vi "Curcular Buffer Data History.vi"(6 "Oldest time to Plot":dbl, 7 "write (F)":bool, 8 "Error In":errorcluster, 9 "Data Value":dbl, 10 "Time Stamp":dbl format="%^<%H:%M:%S%4u\n%x>T", 11 "Device Name":string) -> (0 "Error Out":errorcluster, 1 "Latest Timestamp":dbl, 2 "Latest Value":dbl, 3 "Truncated Data History":T1)   [LabVIEW 2014]
uses:
  typedefs/DVR Map Action.ctl
  typedefs/Data History.ctl
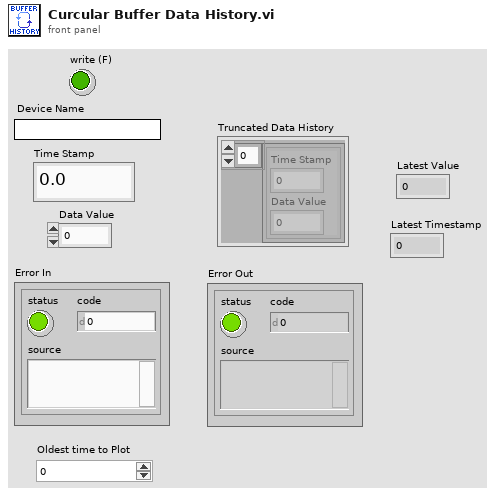
[diagram p1: front panel]
types:
  T1 = cluster{cluster{"Time Stamp":dbl, "Data Value":dbl}[]}
  T2 = typedef "DVR Map Action.ctl" = enum16{"Read Names", "Write", "Read"}
  T3 = typedef "Data History.ctl" = cluster{"Timestamps":dbl[], "Values":dbl[]}
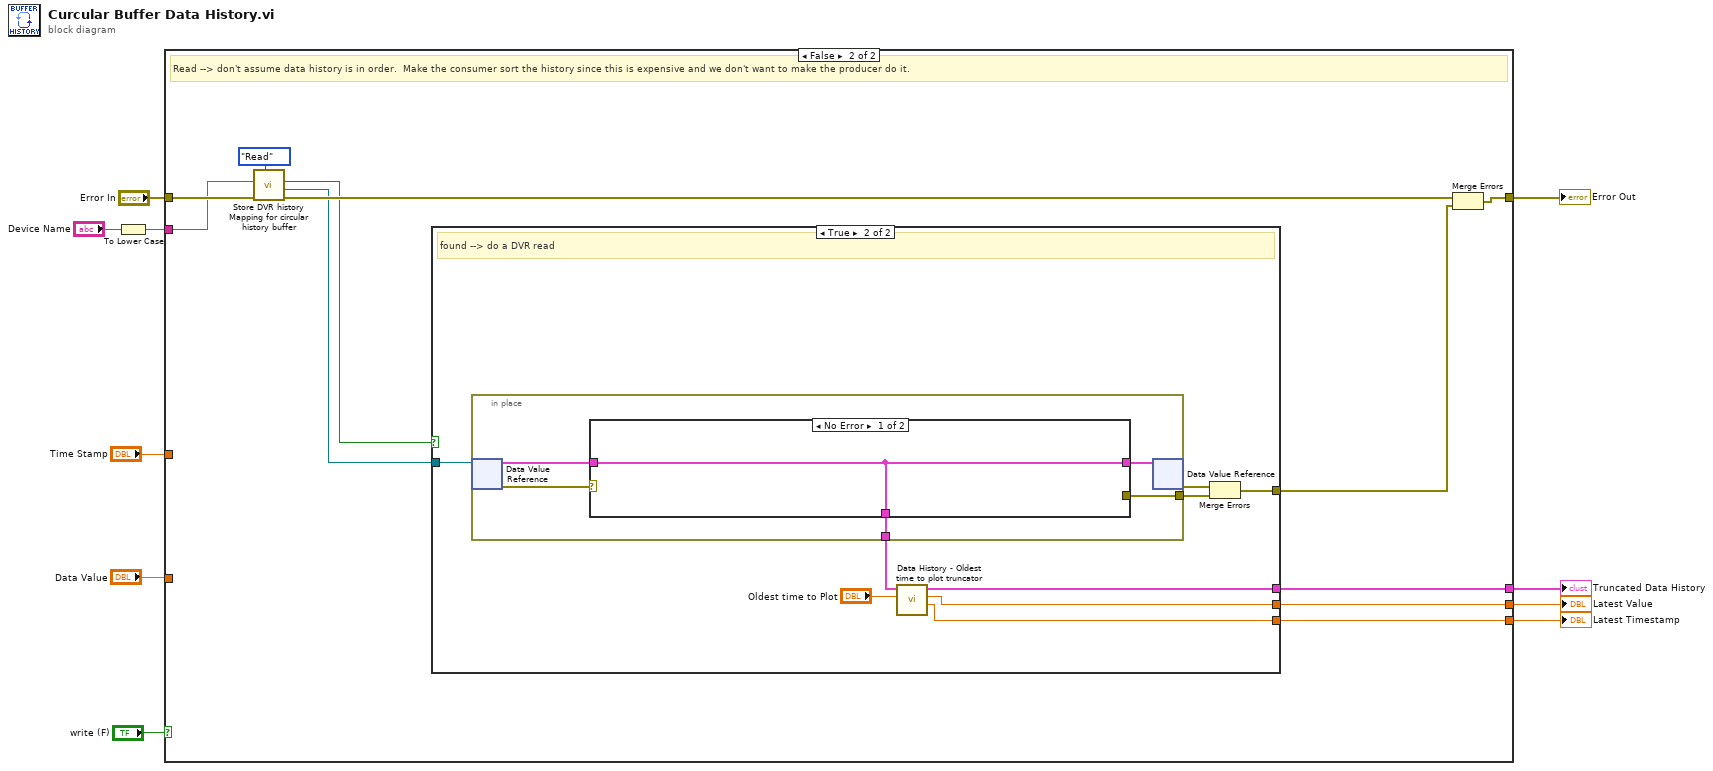
[diagram p0: block diagram]
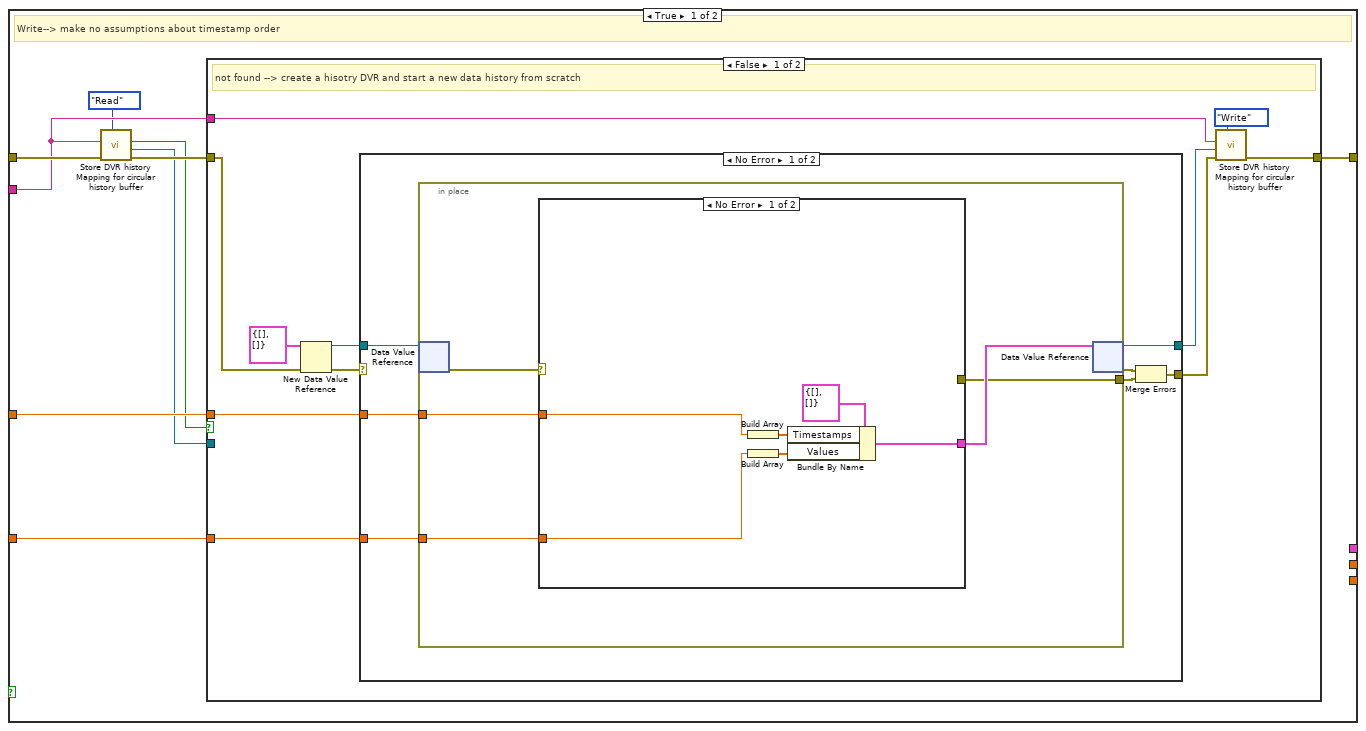
[diagram p2: hidden frame]
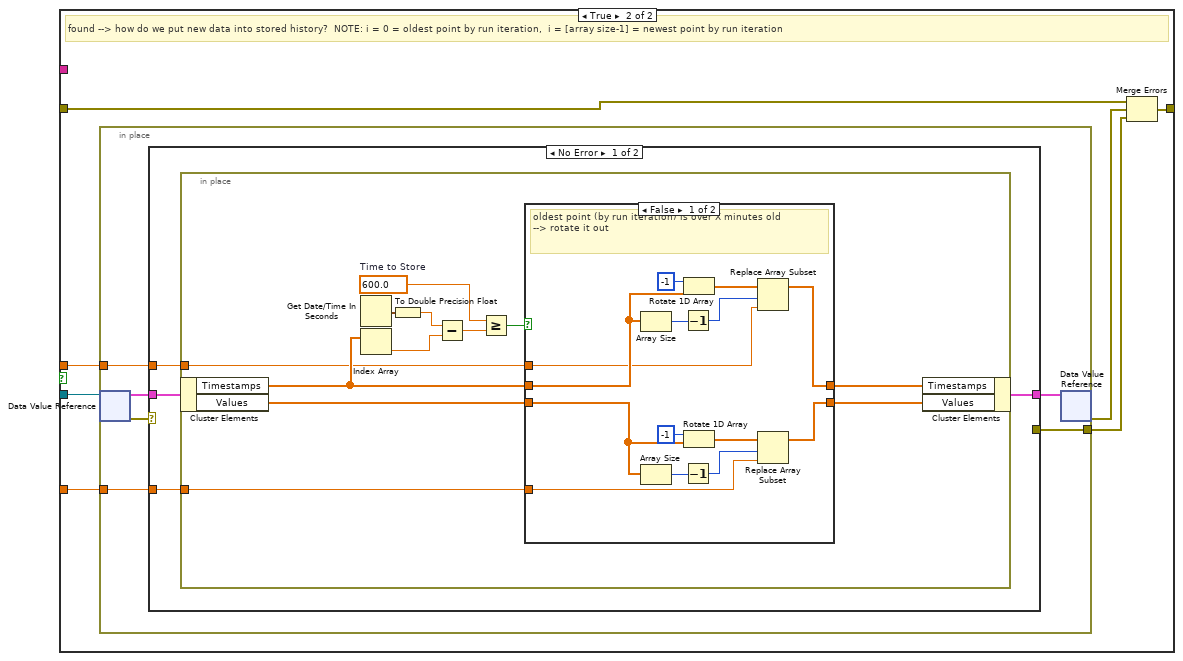
[diagram p5: hidden frame]
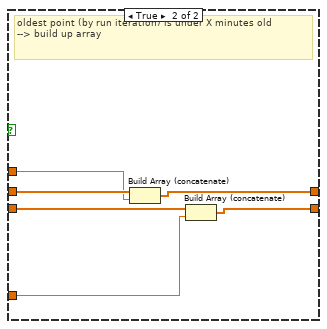
[diagram p6: hidden frame]
diagram:
  n1 = To Lower Case(string="Device Name") -> (all lower case string=w2:string)
  n2 = case shown="False" "write (F)" {
    tunnel: w2 -> [w12 w102]
    tunnel: "Time Stamp" -> [w19 _]
    tunnel: "Data Value" -> [w18 _]
    tunnel: [w17 w110] -> w6
    tunnel: "Error In" -> [w16 w106]
    tunnel: [_ w109] -> w3
    tunnel: [_ w108] -> w5
    tunnel: [_ w107] -> w4
    frame True {
      # "Write--> make no assumptions about timestamp order"
      n3 = call "Store DVR history Mapping for circular history buffer.vi"("Action"=DVR_Map_Action."Read", "error in"=w16, "Device Name"=w12) -> ("error out"=w15:errorcluster, "History DVR"=w13:refnum<data-value>, "Found?"=w14:bool)  [unwired: 5 in, 1 out]
      n4 = case shown="False" w14 {
        tunnel: w13 -> [_ w55]
        tunnel: w19 -> [w30 w57]
        tunnel: w18 -> [w29 w56]
        tunnel: w12 -> [w21 _]
        tunnel: w15 -> [w26 w51]
        tunnel: [w23 w54] -> w17
        frame False {
          # "not found --> create a hisotry DVR and start a new data history from scratch"
          n5 = New Data Value Reference(data value=T3 {"Timestamps"=[], "Values"=[]} ("Current Value Data"), error in=w26) -> (data value reference=w27:refnum<data-value>, error out=w25:errorcluster)
          n6 = case shown="No Error" w25 {
            selector: w25 -> [_ w50]
            tunnel: w30 -> [w37 _]
            tunnel: w29 -> [w36 _]
            tunnel: w27 -> [w35 _]
            tunnel: [w32 w50] -> w24
            tunnel: [w31 _] -> w22
            frame No Error {
              n7 = in-place {
                in-place-border: w37 -> [w42]
                in-place-border: w36 -> [w41]
                in-place-border: [w38] -> w33
                n8 = in-place-dvr #1(w35) -> (w40:errorcluster)  [unwired: 1 out]
                n9 = case shown="No Error" w40 {
                  selector: w40 -> [_ w49]
                  tunnel: w42 -> [w47 _]
                  tunnel: w41 -> [w46 _]
                  tunnel: [w43 _] -> w39
                  tunnel: [_ w49] -> w38
                  frame No Error {
                    n10 = Build Array(w47) -> (w45:dbl[])
                    n11 = Build Array(w46) -> (w44:dbl[])
                    n12 = Bundle By Name(cluster=T3 {"Timestamps"=[], "Values"=[]} ("Current Value Data"), "Timestamps"=w45, "Values"=w44) -> (w43:T3)
                  }
                  frame Error {
                  }
                }
                n13 = in-place-dvr #1(w39) -> (w31:refnum<data-value>, w34:errorcluster)
              }
              n14 = Merge Errors(w34, w33) -> (w32:errorcluster)
            }
            frame Error {
            }
          }
          n15 = call "Store DVR history Mapping for circular history buffer.vi"("Action"=DVR_Map_Action."Write", "error in"=w24, "History DVR"=w22, "Device Name"=w21) -> ("error out"=w23:errorcluster)  [unwired: 4 in, 3 out]
        }
        frame True {
          # "found --> how do we put new data into stored history?  NOTE: i = 0 = oldest point by run iteration,  i = [array size-1] = newest point by run iteration"
          n16 = in-place {
            in-place-border: w57 -> [w62]
            in-place-border: w56 -> [w63]
            in-place-border: [w58] -> w53
            n17 = in-place-dvr #2(w55) -> (w60:T3, w61:errorcluster)
            n18 = case shown="No Error" w61 {
              selector: w61 -> [_ w100]
              tunnel: w63 -> [w67 _]
              tunnel: w62 -> [w66 _]
              tunnel: w60 -> [w65 _]
              tunnel: [w64 _] -> w59
              tunnel: [_ w100] -> w58
              frame No Error {
                n19 = in-place {
                  in-place-border: w67 -> [w79]
                  in-place-border: w66 -> [w73]
                  w71 = 600.0  # Time to Store
                  n20 = in-place-cluster #3(w65) -> ("Timestamps"=w78:dbl[], "Values"=w77:dbl[])
                  n21 = Get Date/Time In Seconds() -> (seconds since 1Jan1904=w74:timestamp)
                  n22 = Index Array(array=w78) -> (element=w70:dbl)  [unwired: 1 in]
                  n23 = To Double Precision Float(number=w74) -> (double precision float=w72:dbl)
                  n24 = Subtract(x=w72, y=w70) -> (x-y=w69:dbl)
                  n25 = Greater Or Equal?(x=w71, y=w69) -> (x >= y?=w68:bool)
                  n26 = case shown="False" w68 {
                    tunnel: w77 -> [w85 w96]
                    tunnel: w79 -> [w84 w95]
                    tunnel: [w83 w97] -> w76
                    tunnel: [w82 w94] -> w75
                    tunnel: w78 -> [w81 w99]
                    tunnel: w73 -> [w80 w98]
                    frame False {
                      # "oldest point (by run iteration) is over X minutes old\n--> rotate it out"
                      n27 = Array Size(array=w81) -> (size(s)=w90:i32)
                      n28 = Array Size(array=w85) -> (size(s)=w89:i32)
                      n29 = Decrement(x=w90) -> (x-1=w93:i32)
                      n30 = Decrement(x=w89) -> (x-1=w86:i32)
                      n31 = Rotate 1D Array(1:w81, 2:-1 ("n")) -> (0:w92:dbl[])
                      n32 = Rotate 1D Array(1:w85, 2:-1 ("n")) -> (0:w87:dbl[])
                      n33 = Replace Array Subset(array=w92, new element=w80, index=w93) -> (w83:dbl[])
                      n34 = Replace Array Subset(array=w87, new element=w84, index=w86) -> (w82:dbl[])
                    }
                    frame True {
                      # "oldest point (by run iteration) is under X minutes old\n--> build up array"
                      n35 = Build Array (concatenate)(w99, w98) -> (w97:dbl[])
                      n36 = Build Array (concatenate)(w96, w95) -> (w94:dbl[])
                    }
                  }
                  n37 = in-place-cluster #3("Timestamps"=w76, "Values"=w75) -> (w64:T3)
                }
              }
              frame Error {
              }
            }
            n38 = in-place-dvr #2(w59) -> (w52:errorcluster)  [unwired: 1 out]
          }
          n39 = Merge Errors(w51, w52, w53) -> (w54:errorcluster)
        }
      }
    }
    frame False {
      # "Read --> don't assume data history is in order.  Make the consumer sort the history since this is expensive and we don't want to make the producer do it."
      n40 = call "Store DVR history Mapping for circular history buffer.vi"("Action"=DVR_Map_Action."Read", "error in"=w106, "Device Name"=w102) -> ("error out"=w105:errorcluster, "History DVR"=w104:refnum<data-value>, "Found?"=w103:bool)  [unwired: 5 in, 1 out]
      n41 = case shown="True" w103 {
        tunnel: w104 -> [_ w120]
        tunnel: [_ w117] -> w111
        tunnel: [_ w115] -> w109
        tunnel: [_ w113] -> w108
        tunnel: [_ w114] -> w107
        frame False {
          # "not found --> return empty data"
        }
        frame True {
          # "found --> do a DVR read"
          n42 = in-place {
            in-place-border: [w122] -> w118
            in-place-border: [w121] -> w112
            n43 = in-place-dvr #4(w120) -> (w124:T3, w125:errorcluster)
            n44 = case shown="No Error" w125 {
              selector: w125 -> [_ w127]
              tunnel: w124 -> [w126 w128]
              tunnel: [w126 w128] -> w123
              tunnel: [_ w127] -> w122
              tunnel: [w126 _] -> w121
              frame No Error {
              }
              frame Error {
              }
            }
            n45 = in-place-dvr #4(w123) -> (w119:errorcluster)  [unwired: 1 out]
          }
          n46 = call "Data History - Oldest time to plot truncator.vi"("Oldest Time To Plot"="Oldest time to Plot", "Full History Data"=w112) -> ("Latest Timestamp"=w114:dbl, "Latest Value"=w113:dbl, "Truncated Data History"=w115:T1)  [unwired: 7 in]
          n47 = Merge Errors(w119, w118) -> (w117:errorcluster)
        }
      }
      n48 = Merge Errors(w105, w111) -> (w110:errorcluster)
    }
  }
  "Error Out" <- w6
  "Latest Value" <- w5
  "Latest Timestamp" <- w4
  "Truncated Data History" <- w3
